vi "stop.vi"(3 "error in (no error)":errorcluster, 4 "stop":bool, 5 "niDAQmxAO in":refnum<class "niDAQmxAO.lvclass">) -> (0 "error out":errorcluster, 1 "Stopped":bool, 2 "niDAQmxAO out":refnum<class "niDAQmxAO.lvclass">)   [LabVIEW 2011, in "Hardware.lvlib" / "Channels.lvlib" / "niDAQmxAO.lvclass"]
uses:
  niDAQmxAO.lvclass
  C:/Program Files/National Instruments/LabVIEW 2011/resource/objmgr/daqmx.rc
panel:
  out "SampQuant.SampPerChan":dbl
  out "TotalSampPerChanGenerated":dbl
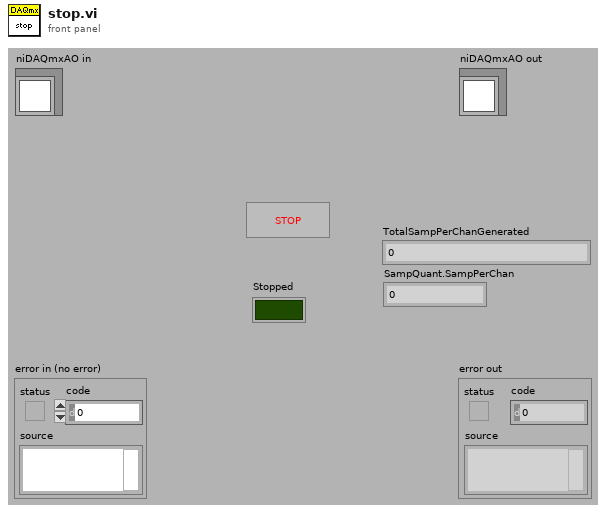
[diagram p1: front panel]
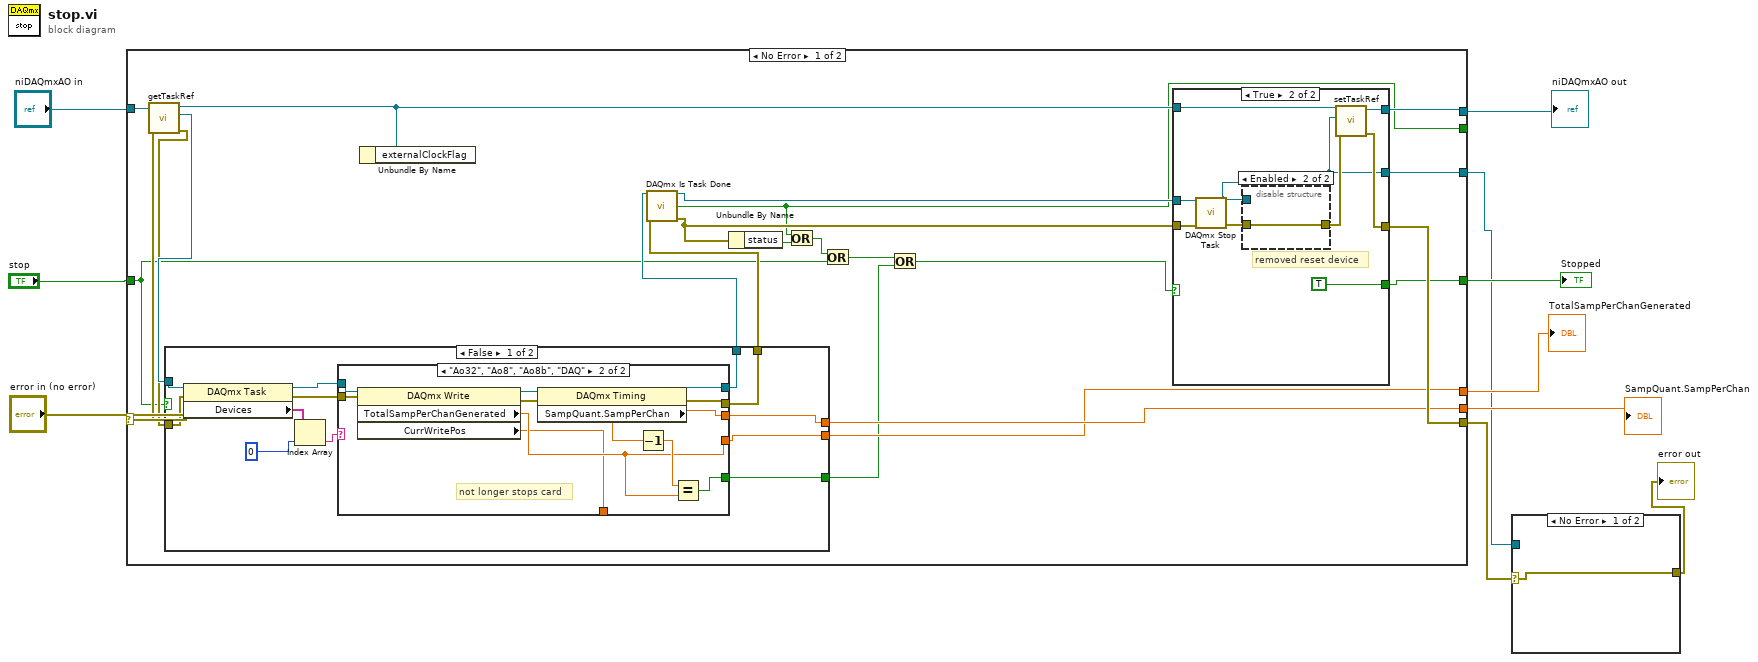
[diagram p0: block diagram]
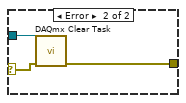
[diagram p2: hidden frame]
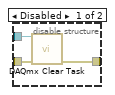
[diagram p6: hidden frame]
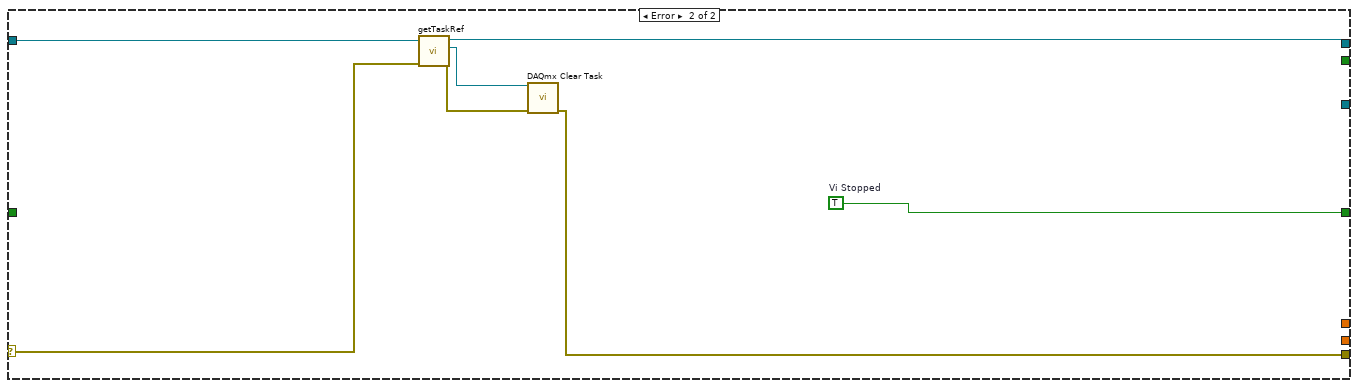
[diagram p7: hidden frame]
diagram:
  n1 = case shown="No Error" "error in (no error)" {
    selector: "error in (no error)" -> [w31 w82]
    tunnel: [w28 w78] -> w2
    tunnel: [w18 w79] -> w8
    tunnel: "niDAQmxAO in" -> [w32 w83]
    tunnel: "stop" -> [w15 _]
    tunnel: [w25 w77] -> w6
    tunnel: [w17 _] -> _
    tunnel: [w20 _] -> w5
    tunnel: [w21 _] -> w4
    tunnel: [w11 _] -> w3
    frame No Error {
      n2 = call "getTaskRef.vi"("error in (no error)"=w31, "niDAQmxAO.lvclass in"=w32) -> ("error out"=w23:errorcluster, "DAQmx Task Ref"=w24:refnum<k21>, "niDAQmxAO.lvclass out"=w19:refnum<class "niDAQmxAO.lvclass">)  [unwired: 7 in]
      n3 = case shown="False" w15 {
        tunnel: w24 -> [w41 w59]
        tunnel: w23 -> [w40 w58]
        tunnel: [w44 w59] -> w22
        tunnel: [w43 w58] -> w16
        tunnel: [w34 _] -> w21
        tunnel: [w42 _] -> w20
        tunnel: [w33 _] -> w13
        frame False {
          n4 = property class="DAQmx Task"(reference=w41, error in=w40) -> (reference out=w39:refnum<k21>, error out=w38:errorcluster, "Devices"=w36:tag[])
          n5 = Index Array(array=w36, index=0) -> (element=w35:tag)
          n6 = case shown="\"Ao32\", \"Ao8\", \"Ao8b\", \"DAQ\"" w35 {
            tunnel: [w46 w52] -> w44
            tunnel: [w45 w55] -> w43
            tunnel: [_ w49] -> w42
            tunnel: w39 -> [w46 w54]
            tunnel: w38 -> [w45 w53]
            tunnel: [_ w51] -> w34
            tunnel: [_ w48] -> w33
            tunnel: [_ w47] -> _
            frame Default {
            }
            frame "Ao32", "Ao8", "Ao8b", "DAQ" {
              # "not longer stops card"
              n7 = property class="DAQmx Write"(reference=w54, error in=w53) -> (reference out=w57:refnum<k21>, error out=w56:errorcluster, "TotalSampPerChanGenerated"=w49:dbl, "CurrWritePos"=w47:dbl)
              n8 = property class="DAQmx Timing"(reference=w57, error in=w56) -> (reference out=w52:refnum<k21>, error out=w55:errorcluster, "SampQuant.SampPerChan"=w51:dbl)
              n9 = Decrement(x=w51) -> (x-1=w50:dbl)
              n10 = Equal?(x=w50, y=w49) -> (x = y?=w48:bool)
            }
          }
        }
        frame True {
        }
      }
      n11 = Unbundle By Name(w19) -> ()  [unwired: 1 out]
      n12 = call <vilib>:"DAQmx Is Task Done.vi"("task/channels in"=w22, "error in"=w16) -> ("task out"=w30:refnum<k21>, "task done?"=w17:bool, "error out"=w29:errorcluster)  [unwired: 11 in]
      n13 = Unbundle By Name(w29) -> ("status"=w26:bool)
      n14 = Or(x=w17, y=w26) -> (x .or. y?=w27:bool)
      n15 = Or(x=w27, y=w15) -> (x .or. y?=w14:bool)
      n16 = Or(x=w14, y=w13) -> (x .or. y?=w12:bool)
      n17 = case shown="True" w12 {
        selector: w12 -> [w62 _]
        tunnel: w30 -> [w60 w70]
        tunnel: w29 -> [w63 w71]
        tunnel: [w63 w68] -> w28
        tunnel: [w62 TRUE] -> w25
        tunnel: w19 -> [w61 w69]
        tunnel: [w61 w67] -> w18
        tunnel: [w60 w64] -> w11
        frame False {
        }
        frame True {
          # "removed reset device"
          n18 = call <vilib>:"DAQmx Stop Task.vi"("task/channels in"=w70, "error in"=w71) -> ("task out"=w64:refnum<k21>, "error out"=w66:errorcluster)  [unwired: 12 in]
          n19 = disable-structure shown="Enabled" {
            disable-tunnel: w66 -> [w75 w76]
            disable-tunnel: [w74 w76] -> w65
            disable-tunnel: w64 -> [w73 _]
            frame Disabled {
              n20 = call <vilib>:"DAQmx Clear Task.vi"("task in"=w73, "error in"=w75) -> ("error out"=w74:errorcluster)  [unwired: 13 in]
            }
            frame Enabled {
            }
          }
          n21 = call "setTaskRef.vi"("error in (no error)"=w65, "DAQmx Task Ref"=w64, "niDAQmxAO.lvclass in"=w69) -> ("error out"=w68:errorcluster, "niDAQmxAO.lvclass out"=w67:refnum<class "niDAQmxAO.lvclass">)  [unwired: 7 in]
        }
      }
    }
    frame Error {
      w77 = TRUE  # Vi Stopped
      n22 = call "getTaskRef.vi"("error in (no error)"=w82, "niDAQmxAO.lvclass in"=w83) -> ("error out"=w80:errorcluster, "DAQmx Task Ref"=w81:refnum<k21>, "niDAQmxAO.lvclass out"=w79:refnum<class "niDAQmxAO.lvclass">)  [unwired: 7 in]
      n23 = call <vilib>:"DAQmx Clear Task.vi"("task in"=w81, "error in"=w80) -> ("error out"=w78:errorcluster)  [unwired: 13 in]
    }
  }
  "niDAQmxAO out" <- w8
  "Stopped" <- w6
  "TotalSampPerChanGenerated" <- w5
  "SampQuant.SampPerChan" <- w4
  n24 = case shown="No Error" w2 {
    selector: w2 -> [w84 w86]
    tunnel: w3 -> [_ w87]
    tunnel: [w84 w85] -> w1
    frame No Error {
    }
    frame Error {
      n25 = call <vilib>:"DAQmx Clear Task.vi"("task in"=w87, "error in"=w86) -> ("error out"=w85:errorcluster)  [unwired: 13 in]
    }
  }
  "error out" <- w1
